vi "acceptStartCommand.vi"(8 "error in (no error)":errorcluster, 11 "SALCommunicator in":refnum<class "SALCommunicatorDL.lvclass">) -> (0 "error out":errorcluster, 1 "configuration":string, 2 "Command ID":i32, 3 "SALCommunicator out":refnum<class "SALCommunicatorDL.lvclass">)   [LabVIEW 2016, in "SALCommunicatorDL.lvclass"]
uses:
  SALCommunicatorDL.lvclass
  ts_sallv_exa/SALLV_EXA.lvlib
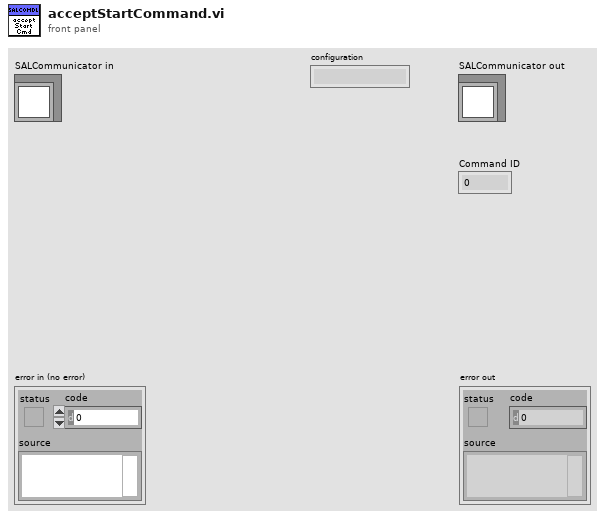
[diagram p1: front panel]
types:
  T1 = typedef "SALLV_EXA.lvlib/command_start.ctl" = cluster{"configuration":string}
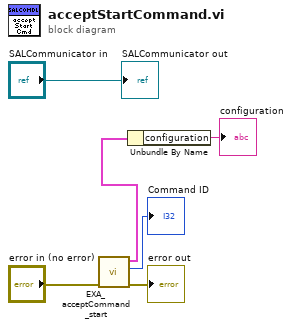
[diagram p0: block diagram]
diagram:
  n1 = call "EXA_acceptCommand_start.vi"("error in (no error)"="error in (no error)") -> ("error out"=→"error out":errorcluster, "function return"=→"Command ID":i32, "command_start_Ctl out"=w2:T1)  [unwired: 8 in]
  n2 = Unbundle By Name(w2) -> ("configuration"=→"configuration":string)
  "SALCommunicator out" <- "SALCommunicator in"
